vi "treadmill_main.vi"() -> ()   [LabVIEW 2018]
uses:
  #typedef_DefinedStates.ctl
  SpeedAndTimeCluster.ctl
  FollowingSteps.ctl
  OperateCluster.ctl
panel:
  out "Speed":u16
  out "Time":u16
  in  "Slower":bool
  in  "Faster":bool
  in  "Exit":bool
  in  "QuickStart":bool
  in  "Start Program":bool
  in  "DefineProg":bool
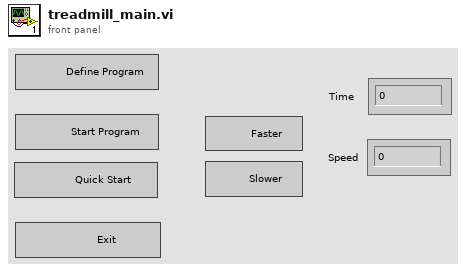
[diagram p1: front panel]
types:
  T1 = typedef "OperateCluster.ctl" = cluster{"SpeedAndTime":T2, "Following Steps":T3, "CurrentStep 2":T2, "Coutnter":u16, "WorkStepsCoutner":u16, "LastIndex":i32, "LastState":T4}
  T2 = typedef "SpeedAndTimeCluster.ctl" = cluster{"Time ":u16, " Speed":u16}
  T3 = typedef "FollowingSteps.ctl" = T2[]
  T4 = typedef "#typedef_DefinedStates.ctl" = enum16{"Init", "Config", "DefineProgram", "StartProgram", "WorkAsUWant", "ChangeStep", "WorkwithSteps", "ExitProgram"}
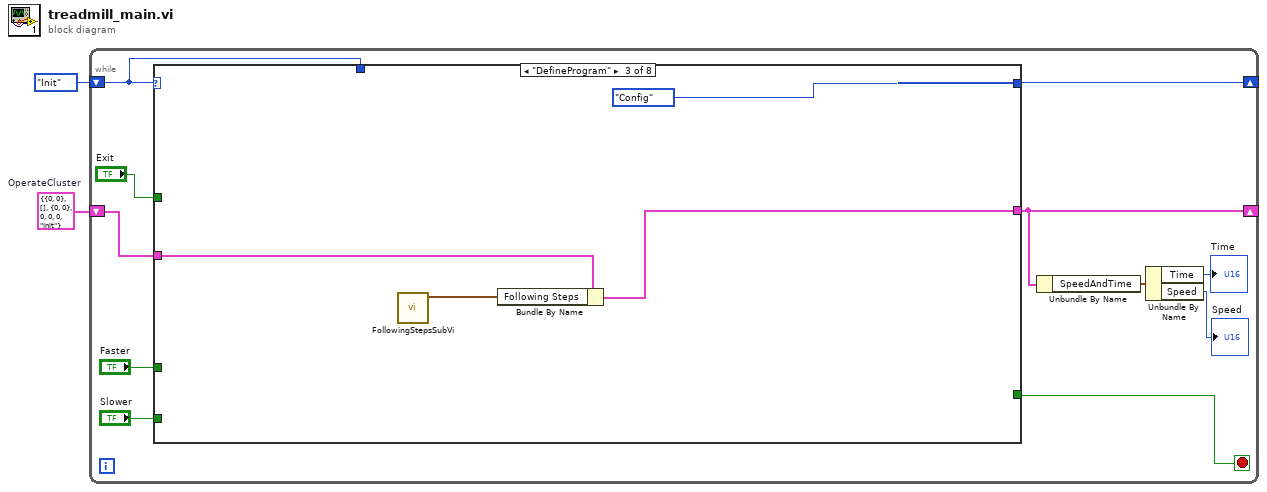
[diagram p0: block diagram]
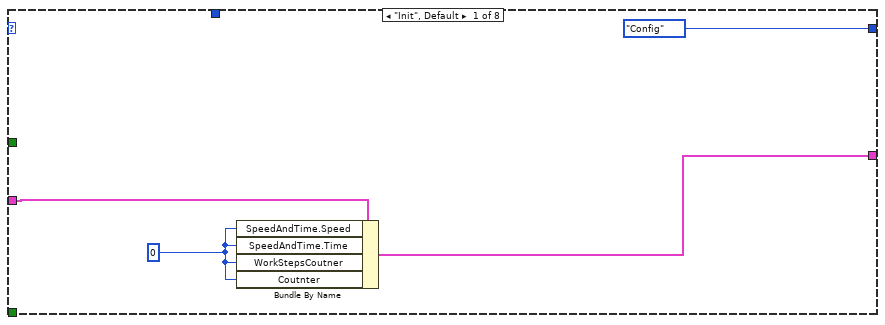
[diagram p2: hidden frame]
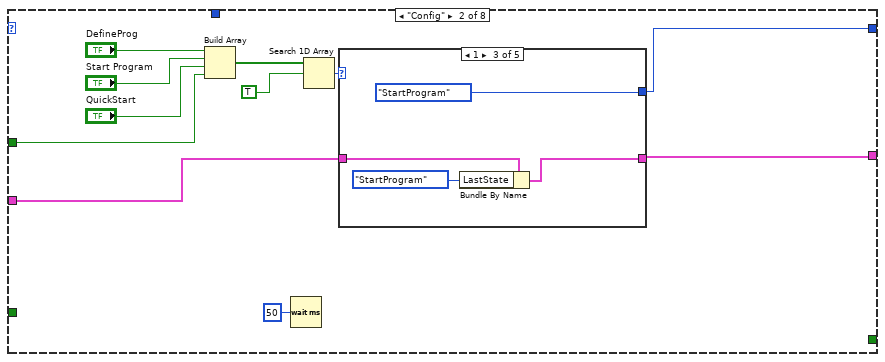
[diagram p3: hidden frame]
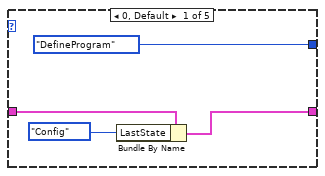
[diagram p4: hidden frame]
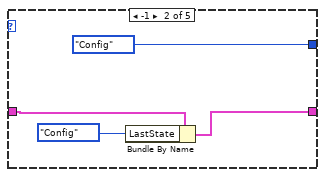
[diagram p5: hidden frame]
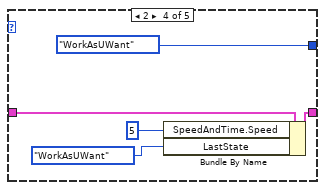
[diagram p6: hidden frame]
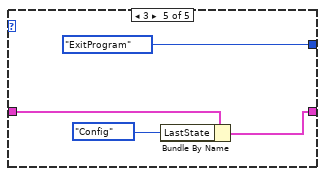
[diagram p7: hidden frame]
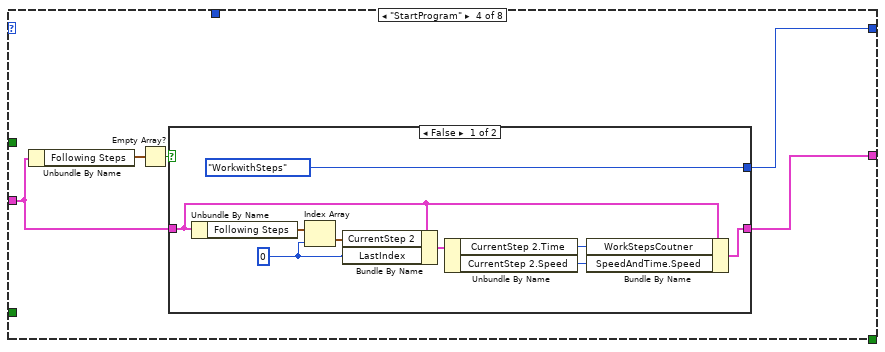
[diagram p8: hidden frame]
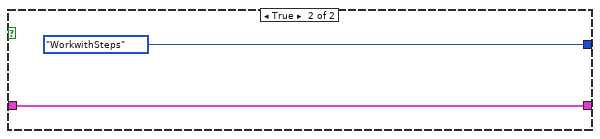
[diagram p9: hidden frame]
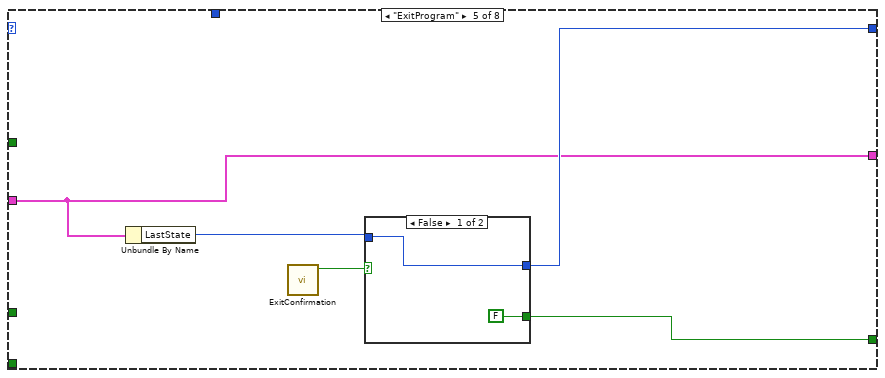
[diagram p10: hidden frame]
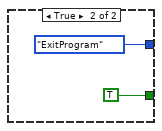
[diagram p11: hidden frame]
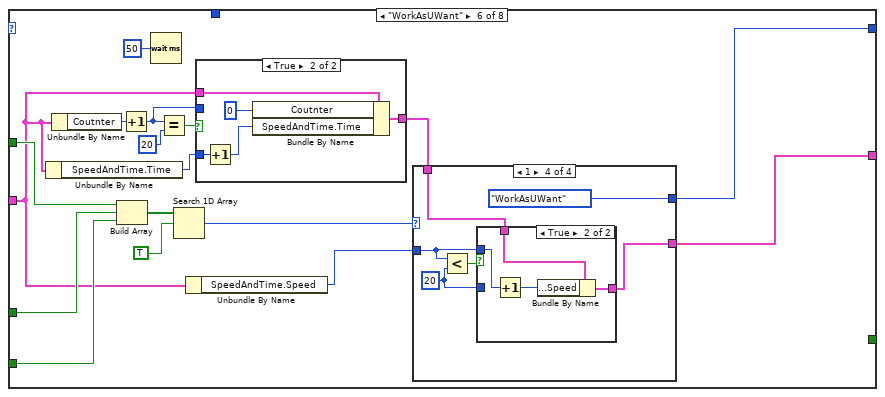
[diagram p12: hidden frame]
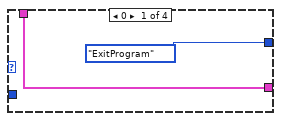
[diagram p13: hidden frame]
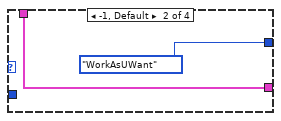
[diagram p14: hidden frame]
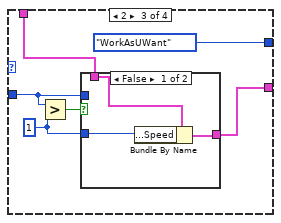
[diagram p15: hidden frame]
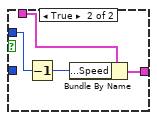
[diagram p16: hidden frame]
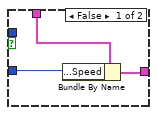
[diagram p17: hidden frame]
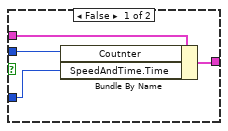
[diagram p18: hidden frame]
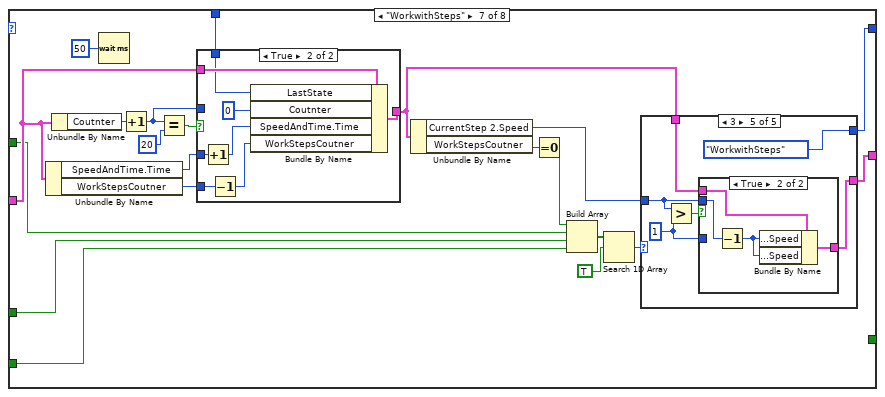
[diagram p19: hidden frame]
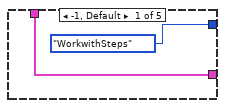
[diagram p20: hidden frame]
diagram:
  w1 = T1 {"SpeedAndTime"={"Time "=0, " Speed"=0}, "Following Steps"=[], "CurrentStep 2"={"Time "=0, " Speed"=0}, "Coutnter"=0, "WorkStepsCoutner"=0, "LastIndex"=0, "LastState"=enum."Init"}  # OperateCluster
  n1 = while {
    shift-right: [w11] -> _
    shift-left: #typedef_DefinedStates."Init" -> [w3]
    shift-right: [w9] -> _
    shift-left: w1 -> [w10]
    stop <- w4 stop-if-true
    n2 = case shown="\"DefineProgram\"" w3 {
      tunnel: [#typedef_DefinedStates."Config" w20 #typedef_DefinedStates."Config" w56 w73 w83 w137 w201] -> w11
      tunnel: w10 -> [w16 w23 w51 w55 w71 w80 w145 w204]
      tunnel: [w15 w22 w50 w54 w71 w81 w138 w207] -> w9
      tunnel: "Faster" -> [_ _ _ _ _ w94 w143 _]
      tunnel: "Slower" -> [_ _ _ _ _ w93 w144 _]
      tunnel: "Exit" -> [_ w19 _ _ _ w85 w141 _]
      tunnel: [_ _ _ _ w72 _ _ _] -> w4
      tunnel: w3 -> [_ _ _ _ _ _ w136 _]
      frame "Init", Default {
        w14 = u16 0 ("index")
        n3 = Bundle By Name(cluster=w16, "SpeedAndTime.Speed"=w14, "SpeedAndTime.Time"=w14, "WorkStepsCoutner"=w14, "Coutnter"=w14) -> (w15:T1)
      }
      frame "Config" {
        n4 = Build Array("DefineProg", "Start Program", "QuickStart", w19) -> (w25:bool[])
        n5 = Wait (ms)(milliseconds to wait=u32 50) -> ()  [unwired: 1 out]
        n6 = Search 1D Array(1D array=w25, element=TRUE) -> (index of element=w24:i32)  [unwired: 1 in]
        n7 = case shown="1" w24 {
          tunnel: [#typedef_DefinedStates."DefineProgram" #typedef_DefinedStates."Config" #typedef_DefinedStates."StartProgram" #typedef_DefinedStates."WorkAsUWant" #typedef_DefinedStates."ExitProgram"] -> w20
          tunnel: w23 -> [w31 w34 w38 w45 w47]
          tunnel: [w30 w33 w37 w44 w46] -> w22
          frame 0, Default {
            n8 = Bundle By Name(cluster=w31, "LastState"=#typedef_DefinedStates."Config") -> (w30:T1)
          }
          frame -1 {
            n9 = Bundle By Name(cluster=w34, "LastState"=#typedef_DefinedStates."Config") -> (w33:T1)
          }
          frame 1 {
            n10 = Bundle By Name(cluster=w38, "LastState"=#typedef_DefinedStates."StartProgram") -> (w37:T1)
          }
          frame 2 {
            n11 = Bundle By Name(cluster=w45, "SpeedAndTime.Speed"=u16 5 ("CurrentStep 2. Speed"), "LastState"=#typedef_DefinedStates."WorkAsUWant") -> (w44:T1)
          }
          frame 3 {
            n12 = Bundle By Name(cluster=w47, "LastState"=#typedef_DefinedStates."Config") -> (w46:T1)
          }
        }
      }
      frame "DefineProgram" {
        n13 = call "FollowingStepsSubVi.vi"() -> ("ArrayOutput"=w52:T3)  [unwired: 11 in]
        n14 = Bundle By Name(cluster=w51, "Following Steps"=w52) -> (w50:T1)
      }
      frame "StartProgram" {
        n15 = Unbundle By Name(w55) -> ("Following Steps"=w58:T3)
        n16 = Empty Array?(array=w58) -> (empty?=w57:bool)
        n17 = case shown="False" w57 {
          tunnel: [#typedef_DefinedStates."WorkwithSteps" #typedef_DefinedStates."WorkwithSteps"] -> w56
          tunnel: w55 -> [w61 w68]
          tunnel: [w60 w68] -> w54
          frame False {
            w64 = 0 ("index")
            n18 = Unbundle By Name(w61) -> ("Following Steps"=w66:T3)
            n19 = Index Array(array=w66, index=w64) -> (element=w65:T2)
            n20 = Bundle By Name(cluster=w61, "CurrentStep 2"=w65, "LastIndex"=w64) -> (w63:T1)
            n21 = Unbundle By Name(w63) -> ("CurrentStep 2.Time"=w62:u16, "CurrentStep 2.Speed"=w59:u16)
            n22 = Bundle By Name(cluster=w61, "WorkStepsCoutner"=w62, "SpeedAndTime.Speed"=w59) -> (w60:T1)
          }
          frame True {
          }
        }
      }
      frame "ExitProgram" {
        n23 = Unbundle By Name(w71) -> ("LastState"=w70:T4)
        n24 = call "ExitConfirmation.vi"() -> ("Output"=w74:bool)  [unwired: 11 in]
        n25 = case shown="False" w74 {
          tunnel: [w76 #typedef_DefinedStates."ExitProgram"] -> w73
          tunnel: [FALSE TRUE] -> w72
          tunnel: w70 -> [w76 _]
          frame False {
          }
          frame True {
          }
        }
      }
      frame "WorkAsUWant" {
        n26 = Unbundle By Name(w80) -> ("SpeedAndTime.Time"=w84:u16)
        n27 = Unbundle By Name(w80) -> ("Coutnter"=w92:u16)
        n28 = Build Array(w85, w94, w93) -> (w88:bool[])
        n29 = Increment(x=w92) -> (x+1=w89:u16)
        n30 = Wait (ms)(milliseconds to wait=u32 50) -> ()  [unwired: 1 out]
        n31 = Equal?(x=w89, y=u16 20) -> (x = y?=w90:bool)
        n32 = Search 1D Array(1D array=w88, element=TRUE) -> (index of element=w86:i32)  [unwired: 1 in]
        n33 = Unbundle By Name(w80) -> ("SpeedAndTime.Speed"=w79:u16)
        n34 = case shown="True" w90 {
          tunnel: w89 -> [w127 _]
          tunnel: w80 -> [w128 w134]
          tunnel: w84 -> [w126 w132]
          tunnel: [w129 w130] -> w82
          frame False {
            n35 = Bundle By Name(cluster=w128, "Coutnter"=w127, "SpeedAndTime.Time"=w126) -> (w129:T1)
          }
          frame True {
            n36 = Increment(x=w132) -> (x+1=w131:u16)
            n37 = Bundle By Name(cluster=w134, "Coutnter"=u64 0, "SpeedAndTime.Time"=w131) -> (w130:T1)
          }
        }
        n38 = case shown="1" w86 {
          tunnel: [#typedef_DefinedStates."ExitProgram" #typedef_DefinedStates."WorkAsUWant" #typedef_DefinedStates."WorkAsUWant" #typedef_DefinedStates."WorkAsUWant"] -> w83
          tunnel: w82 -> [w96 w98 w101 w114]
          tunnel: [w96 w98 w102 w113] -> w81
          tunnel: w79 -> [_ _ w100 w115]
          frame 0 {
          }
          frame -1, Default {
          }
          frame 2 {
            w103 = u16 1 ("y")
            n39 = Greater?(x=w100, y=w103) -> (0:w104:bool)
            n40 = case shown="False" w104 {
              tunnel: w101 -> [w108 w111]
              tunnel: w100 -> [_ w110]
              tunnel: [w106 w109] -> w102
              tunnel: w103 -> [w107 _]
              frame False {
                n41 = Bundle By Name(cluster=w108, "SpeedAndTime.Speed"=w107) -> (w106:T1)
              }
              frame True {
                n42 = Decrement(x=w110) -> (x-1=w112:u16)
                n43 = Bundle By Name(cluster=w111, "SpeedAndTime.Speed"=w112) -> (w109:T1)
              }
            }
          }
          frame 1 {
            w116 = u16 20 ("y")
            n44 = Less?(x=w115, y=w116) -> (x < y?=w117:bool)
            n45 = case shown="True" w117 {
              tunnel: w114 -> [w121 w124]
              tunnel: w115 -> [_ w123]
              tunnel: [w119 w122] -> w113
              tunnel: w116 -> [w120 _]
              frame False {
                n46 = Bundle By Name(cluster=w121, "CurrentStep 2.Speed"=w120) -> (w119:T1)
              }
              frame True {
                n47 = Increment(x=w123) -> (x+1=w125:u16)
                n48 = Bundle By Name(cluster=w124, "SpeedAndTime.Speed"=w125) -> (w122:T1)
              }
            }
          }
        }
      }
      frame "WorkwithSteps" {
        n49 = Unbundle By Name(w145) -> ("SpeedAndTime.Time"=w148:u16, "WorkStepsCoutner"=w147:u16)
        n50 = Unbundle By Name(w145) -> ("Coutnter"=w152:u16)
        n51 = Wait (ms)(milliseconds to wait=u32 50) -> ()  [unwired: 1 out]
        n52 = Increment(x=w152) -> (x+1=w149:u16)
        n53 = Equal?(x=w149, y=u16 20) -> (x = y?=w150:bool)
        n54 = case shown="True" w150 {
          tunnel: w149 -> [w190 _]
          tunnel: w145 -> [w191 w200]
          tunnel: w148 -> [w189 w198]
          tunnel: [w192 w196] -> w135
          tunnel: w147 -> [_ w195]
          tunnel: w136 -> [w188 w193]
          frame False {
            n55 = Bundle By Name(cluster=w191, "LastState"=w188, "Coutnter"=w190, "SpeedAndTime.Time"=w189) -> (w192:T1)
          }
          frame True {
            n56 = Increment(x=w198) -> (x+1=w197:u16)
            n57 = Decrement(x=w195) -> (x-1=w194:u16)
            n58 = Bundle By Name(cluster=w200, "LastState"=w193, "Coutnter"=u16 0, "SpeedAndTime.Time"=w197, "WorkStepsCoutner"=w194) -> (w196:T1)
          }
        }
        n59 = Unbundle By Name(w135) -> ("CurrentStep 2.Speed"=w139:u16, "WorkStepsCoutner"=w146:u16)
        n60 = Equal To 0?(x=w146) -> (x = 0?=w142:bool)
        n61 = Build Array(w142, w141, w143, w144) -> (w155:bool[])
        n62 = Search 1D Array(1D array=w155, element=TRUE) -> (index of element=w140:i32)  [unwired: 1 in]
        n63 = case shown="3" w140 {
          tunnel: w139 -> [_ _ w162 _ w176]
          tunnel: w135 -> [w157 w159 w163 w174 w177]
          tunnel: [w157 w159 w161 w174 w175] -> w138
          tunnel: [#typedef_DefinedStates."WorkwithSteps" #typedef_DefinedStates."ChangeStep" #typedef_DefinedStates."WorkwithSteps" #typedef_DefinedStates."ExitProgram" #typedef_DefinedStates."WorkwithSteps"] -> w137
          frame -1, Default {
          }
          frame 0 {
          }
          frame 2 {
            w160 = u16 20 ("y")
            n64 = Less?(x=w162, y=w160) -> (x < y?=w164:bool)
            n65 = case shown="True" w164 {
              tunnel: w163 -> [w168 w171]
              tunnel: w162 -> [_ w170]
              tunnel: [w166 w169] -> w161
              tunnel: w160 -> [w167 _]
              frame False {
                n66 = Bundle By Name(cluster=w168, "SpeedAndTime.Speed"=w167, "CurrentStep 2.Speed"=w167) -> (w166:T1)
              }
              frame True {
                n67 = Increment(x=w170) -> (x+1=w172:u16)
                n68 = Bundle By Name(cluster=w171, "SpeedAndTime.Speed"=w172, "CurrentStep 2.Speed"=w172) -> (w169:T1)
              }
            }
          }
          frame 1 {
          }
          frame 3 {
            w179 = u16 1 ("y")
            n69 = Greater?(x=w176, y=w179) -> (0:w180:bool)
            n70 = case shown="True" w180 {
              tunnel: w177 -> [w183 w186]
              tunnel: w176 -> [_ w185]
              tunnel: [w181 w184] -> w175
              tunnel: w179 -> [w182 _]
              frame False {
                n71 = Bundle By Name(cluster=w183, "SpeedAndTime.Speed"=w182, "CurrentStep 2.Speed"=w182) -> (w181:T1)
              }
              frame True {
                n72 = Decrement(x=w185) -> (x-1=w187:u16)
                n73 = Bundle By Name(cluster=w186, "SpeedAndTime.Speed"=w187, "CurrentStep 2.Speed"=w187) -> (w184:T1)
              }
            }
          }
        }
      }
      frame "ChangeStep" {
        n74 = Unbundle By Name(w204) -> ("Following Steps"=w209:T3, "LastIndex"=w210:i32)
        n75 = Unbundle By Name(w204) -> ("Following Steps"=w205:T3)
        n76 = Increment(x=w210) -> (x+1=w202:i32)
        n77 = Array Size(array=w209) -> (size(s)=w208:i32)
        n78 = Index Array(array=w205, index=w202) -> (element=w203:T2)
        n79 = Less?(x=w208, y=w202) -> (x < y?=w206:bool)
        n80 = case shown="True" w206 {
          tunnel: [w211 w219] -> w207
          tunnel: w204 -> [w218 w221]
          tunnel: w203 -> [w217 _]
          tunnel: w202 -> [w216 _]
          tunnel: [#typedef_DefinedStates."WorkwithSteps" #typedef_DefinedStates."Config"] -> w201
          frame False {
            n81 = Bundle By Name(cluster=w218, "LastIndex"=w216, "CurrentStep 2"=w217) -> (w214:T1)
            n82 = Unbundle By Name(w214) -> ("CurrentStep 2.Speed"=w213:u16, "CurrentStep 2.Time"=w212:u16)
            n83 = Bundle By Name(cluster=w214, "SpeedAndTime.Speed"=w213, "WorkStepsCoutner"=w212) -> (w211:T1)
          }
          frame True {
            n84 = Bundle By Name(cluster=w221, "SpeedAndTime.Speed"=u16 0 ("SpeedAndTime. Speed")) -> (w219:T1)
            n85 = call "EndOfTrain.vi"() -> ()  [unwired: 12 in]
          }
        }
      }
    }
    n86 = Unbundle By Name(w9) -> ("SpeedAndTime"=w8:T2)
    n87 = Unbundle By Name(w8) -> ("Time"=→"Time":u16, "Speed"=→"Speed":u16)
  }
